vi "CD Clean-up.vi"(7 "Card Parameters (in)":T1, 8 "Error (in)":errorcluster, 11 "Device Reference":T3 format="%.0x") -> (0 "Error (out)":errorcluster)   [LabVIEW 2019, in "Ballard Arinc-429 Engine.lvlib"]
uses:
  Ballard Arinc-429 Engine.lvlib
  <vilib>/NI VeriStand/Custom Device API/Custom Device Item Ref.ctl
  RT Controls/Card Parameters.ctl
  Shared/Controls and Global/Initialization Method.ctl
  RT Controls/RT Init States.ctl
  <vilib>/NI VeriStand/Custom Device Tools/Custom Device Utility Library/Custom Device Utility Library.lvlib
  <vilib>/NI_Real-Time Target Support.lvlib
  <vilib>/NI VeriStand/Custom Device API/Custom Device API.lvlib
  Shared/Ballard Arinc-429 Shared.lvlib
panel:
  out "Card Parameters (out)":T1
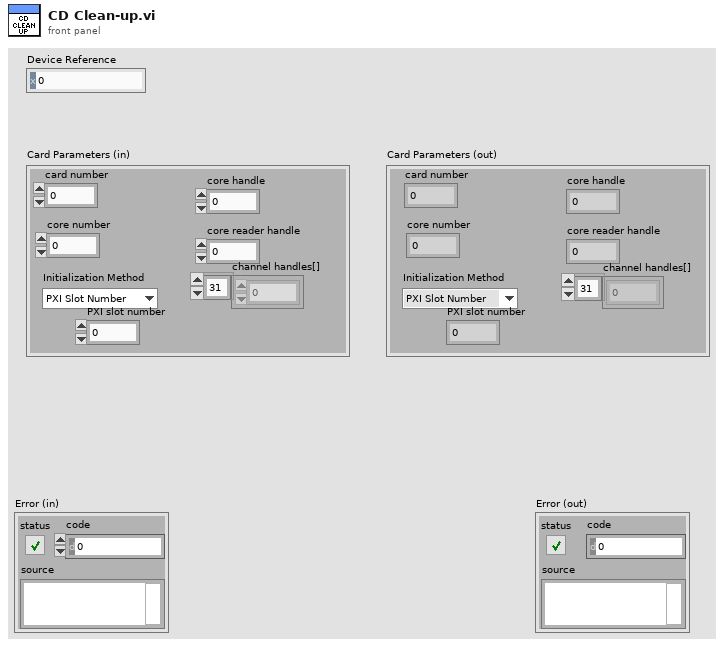
[diagram p1: front panel]
types:
  T1 = typedef "Ballard Arinc-429 Engine.lvlib/Card Parameters.ctl" = cluster{"card number":i32, "core number":i32, "core handle":u64, "core reader handle":u64, "channel handles[]":u64[], "Initialization Method":T2, "PXI slot number":i32}
  T2 = typedef "Ballard Arinc-429 Shared.lvlib/Initialization Method.ctl" = enum16{"PXI Slot Number", "Card Number"}
  T3 = typedef "Custom Device API.lvlib/Custom Device Item Ref.ctl" = u64
  T4 = typedef "Ballard Arinc-429 Engine.lvlib/RT Init States.ctl" = enum16{"Initialization", "Get Card Settings", "Get Channel Count", "Parse Channels", "Ballard-429 Initialize", "Get Status Channels Reference", "Exit"}
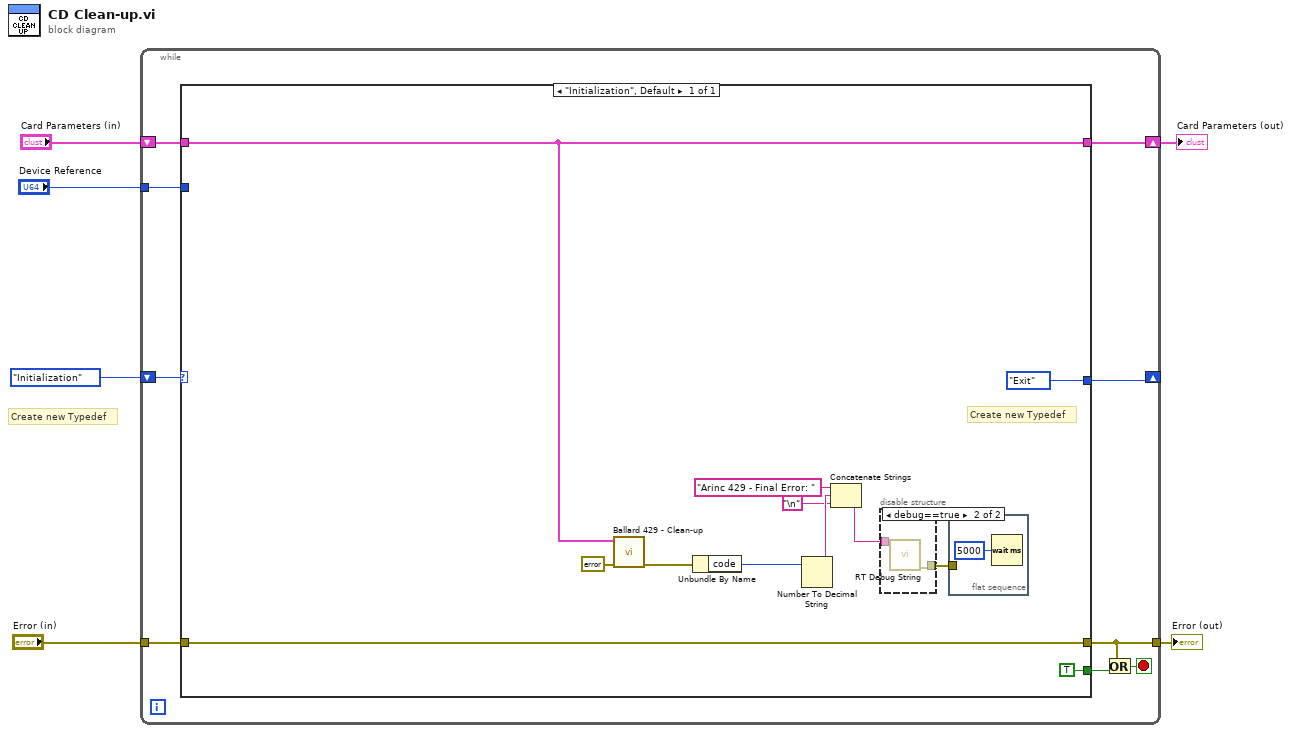
[diagram p0: block diagram]
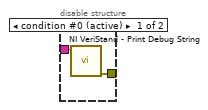
[diagram p2: hidden frame]
diagram:
  # "Create new Typedef"
  n1 = while {
    tunnel: "Error (in)" -> [w14]
    tunnel: [w11] -> w4
    shift-right: [w13] -> _
    shift-left: RT_Init_States."Initialization" -> [w15]
    tunnel: "Device Reference" -> [w12]
    shift-right: [w7] -> w1
    shift-left: "Card Parameters (in)" -> [w8]
    stop <- w10 stop-if-true
    n2 = case shown="\"Initialization\", Default" w15 {
      tunnel: w14 -> [w18]
      tunnel: [w18] -> w11
      tunnel: [RT_Init_States."Exit"] -> w13
      tunnel: w12 -> [_]
      tunnel: [TRUE] -> w9
      tunnel: w8 -> [w25]
      tunnel: [w25] -> w7
      frame "Initialization", Default {
        # "Create new Typedef"
        n3 = call "Ballard 429 - Clean-up.vi"("Error (in)"=errorcluster {"status"=FALSE, "code"=0, "source"=""}, "Card Parameters (in)"=w25) -> ("Error (out)"=w17:errorcluster)  [unwired: 9 in]
        n4 = Unbundle By Name(w17) -> ("code"=w24:i32)
        n5 = Number To Decimal String(number=w24) -> (decimal integer string=w22:string)  [unwired: 1 in]
        n6 = Concatenate Strings("Arinc 429 - Final Error: " ("string"), w22, "\n") -> (w20:string)
        n7 = disable-structure shown="debug==true" {
          disable-tunnel: w20 -> [w29 w31]
          disable-tunnel: [w28 w30] -> w19
          frame condition #0 (active) {
            n8 = call <vilib>:"NI VeriStand - Print Debug String.vi"("Message"=w29) -> ("error out"=w28:errorcluster)  [unwired: 10 in]
          }
          frame condition #1 {
            n9 = call <vilib>:"RT Debug String.vi"("String to write"=w31) -> ("error out"=w30:errorcluster)  [unwired: 10 in]
          }
        }
        n10 = flat-sequence {
          tunnel: w19 -> [_]
          frame #0 {
            n11 = Wait (ms)(milliseconds to wait=u32 5000) -> ()  [unwired: 1 out]
          }
        }
      }
    }
    n12 = Or(x=w11, y=w9) -> (x .or. y?=w10:bool)
  }
  "Error (out)" <- w4
  "Card Parameters (out)" <- w1
